vi "GaitDAQ.vi"() -> ()   [LabVIEW 2019]
panel:
  out "Array 2":u32[][](array[colorbox])
  in  "Array":u32[][](array[colorbox])
  out "Image Number":u32
  in  "Image Logging Prefix":string="Image"
  in  "Image Logging Path":path=path "C:/Users/qiubi/Documents"
  out "Frame Rate":dbl
  in  "Stop (F)":bool
  out "Image Out":T1(plugin-control)
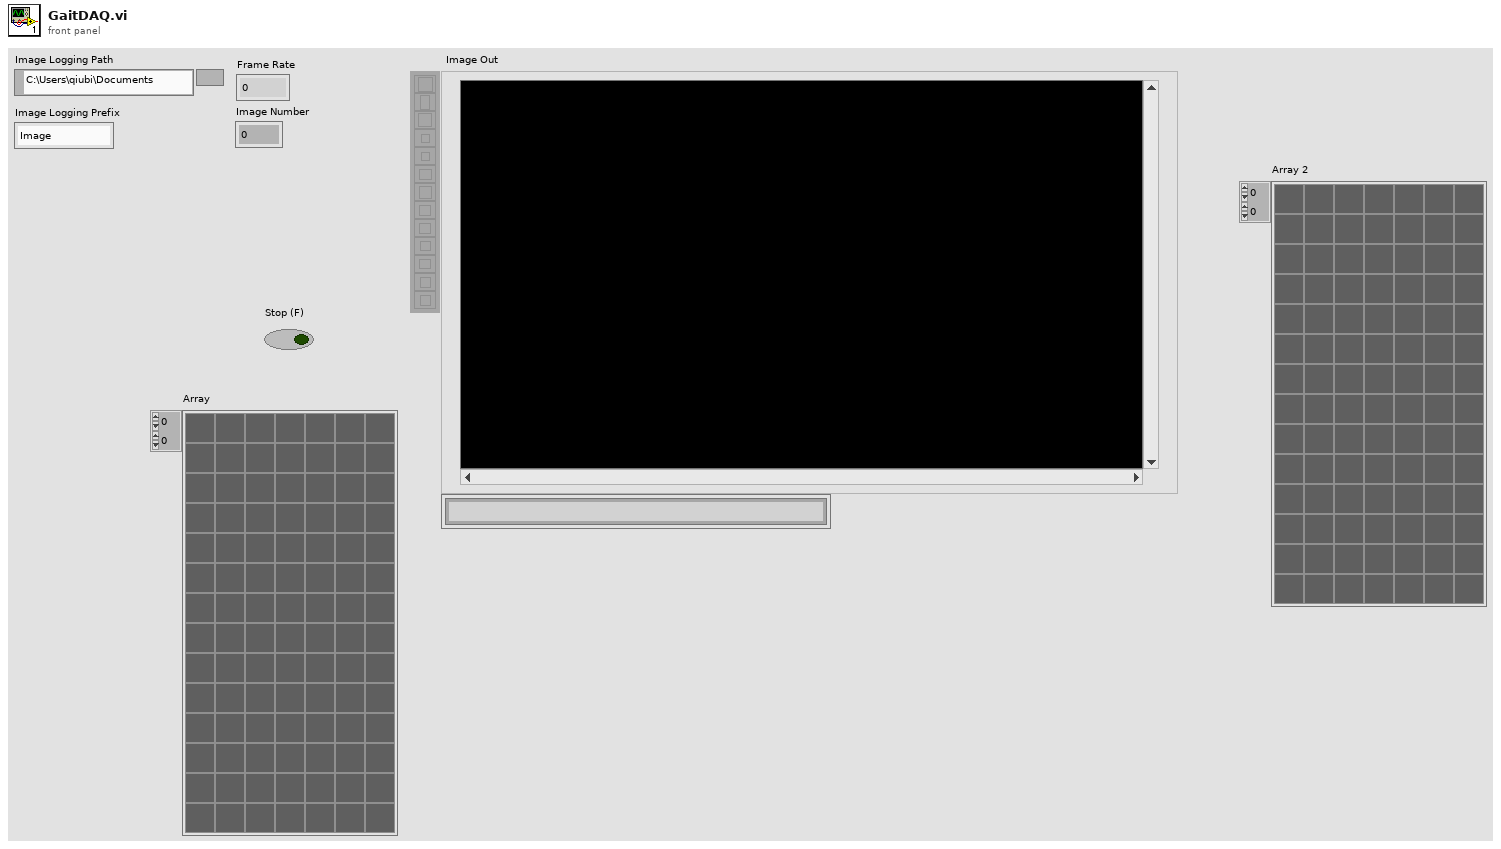
[diagram p1: front panel]
types:
  T1 = typedef "IMAQ Image.ctl" = refnum<image>
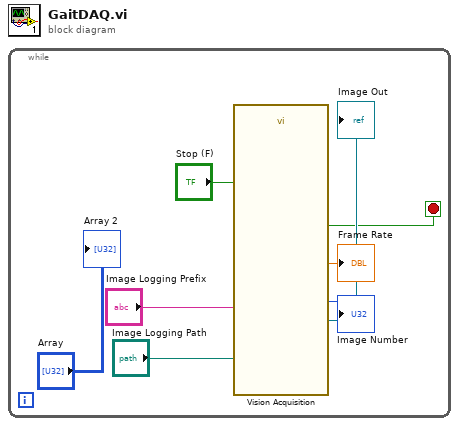
[diagram p0: block diagram]
diagram:
  n1 = while {
    stop <- w6 stop-if-true
    n2 = call "Vision Acquisition"("Image Logging Path"="Image Logging Path", "Image Logging Prefix"="Image Logging Prefix", "Stop (F)"="Stop (F)") -> ("Image Out"=→"Image Out":T1, "Image Number"=→"Image Number":u32, "Frame Rate"=→"Frame Rate":dbl, "Stopped"=w6:bool)  [unwired: 19 in, 2 out]
    "Array 2" <- "Array"
  }
